vi "CreateSignals.vi"(8 "error in (no error)":errorcluster, 11 "DAQList in":refnum<class "DAQList.lvclass">) -> (0 "error out":errorcluster, 2 "Measurement Signals":refnum<k21>[](array[refnum]), 3 "DAQList out":refnum<class "DAQList.lvclass">)   [LabVIEW 2019, in "XCP_DaqDtoId.lvlib" / "DAQList.lvclass"]
uses:
  DAQList.lvclass
  DAQList.lvclass/DAQList.ctl
  <vilib>/ECUMC/ECUMC.llb/MC Get Prop Meas Address.vi
  <vilib>/xnet/xnet.llb/XNET Database Create (Signal).vi
  <vilib>/xnet/xnet.llb/XNET Database Create (Subframe).vi
  <vilib>/Utility/error.llb/Error Cluster From Error Code.vi
  <vilib>/ECUMC/ECUMC.llb/MC Get Prop Meas Data Type.vi
  TypeDef/Global.vi
  <vilib>/xnet/xnet.llb/XNET Database Create (Dynamic Signal).vi
  <vilib>/ECUMC/ECUMC.llb/MC Get Prop Meas Comment.vi
  <vilib>/ECUMC/ECUMC.llb/MC Get Prop Meas Scaling Offset.vi
  <vilib>/ECUMC/ECUMC.llb/MC Get Prop Meas Scaling Factor.vi
  <vilib>/ECUMC/ECUMC.llb/MC Get Prop Meas Minimum.vi
  <vilib>/ECUMC/ECUMC.llb/MC Get Prop Meas Maximum.vi
  <vilib>/ECUMC/ECUMC.llb/MC Get Prop Meas Byte Order.vi
  <vilib>/ECUMC/ECUMC.llb/MC Get Prop Meas Unit.vi
  <vilib>/ErrorRing/Error Ring.xnode
  <resource>/objmgr/xnet.rc
  <vilib>/ECUMC/ECUMC.lvlib
panel:
  out "Previous Offset":i32
  out "Previous Flag":bool
  out "Meas Split Addr Offset":i32
  out "Meas Split Flag":bool
  out "Search Addr":u32 format="%.0x"
  out "Latest Command Pair":u8[][](array[numeric]) format="%.0x"
  in  "For Loop Iteration":i32=-1 caption="#pairs to process (-1 for all)"
  out "Filtered Command Pairs":u8[][][](array[numeric]) format="%.0x"
  # "Debugging Panel"
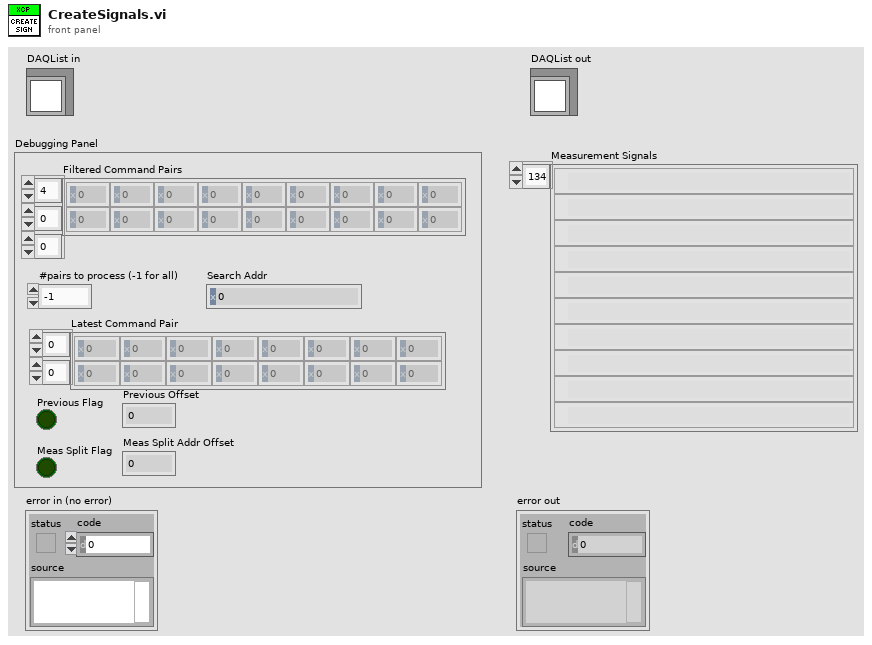
[diagram p1: front panel]
types:
  T1 = typedef "ECUMC.lvlib/MC Reference.ctt" = u32
  T2 = typedef "ECUMC.lvlib/MC Data Type.ctt" = u8
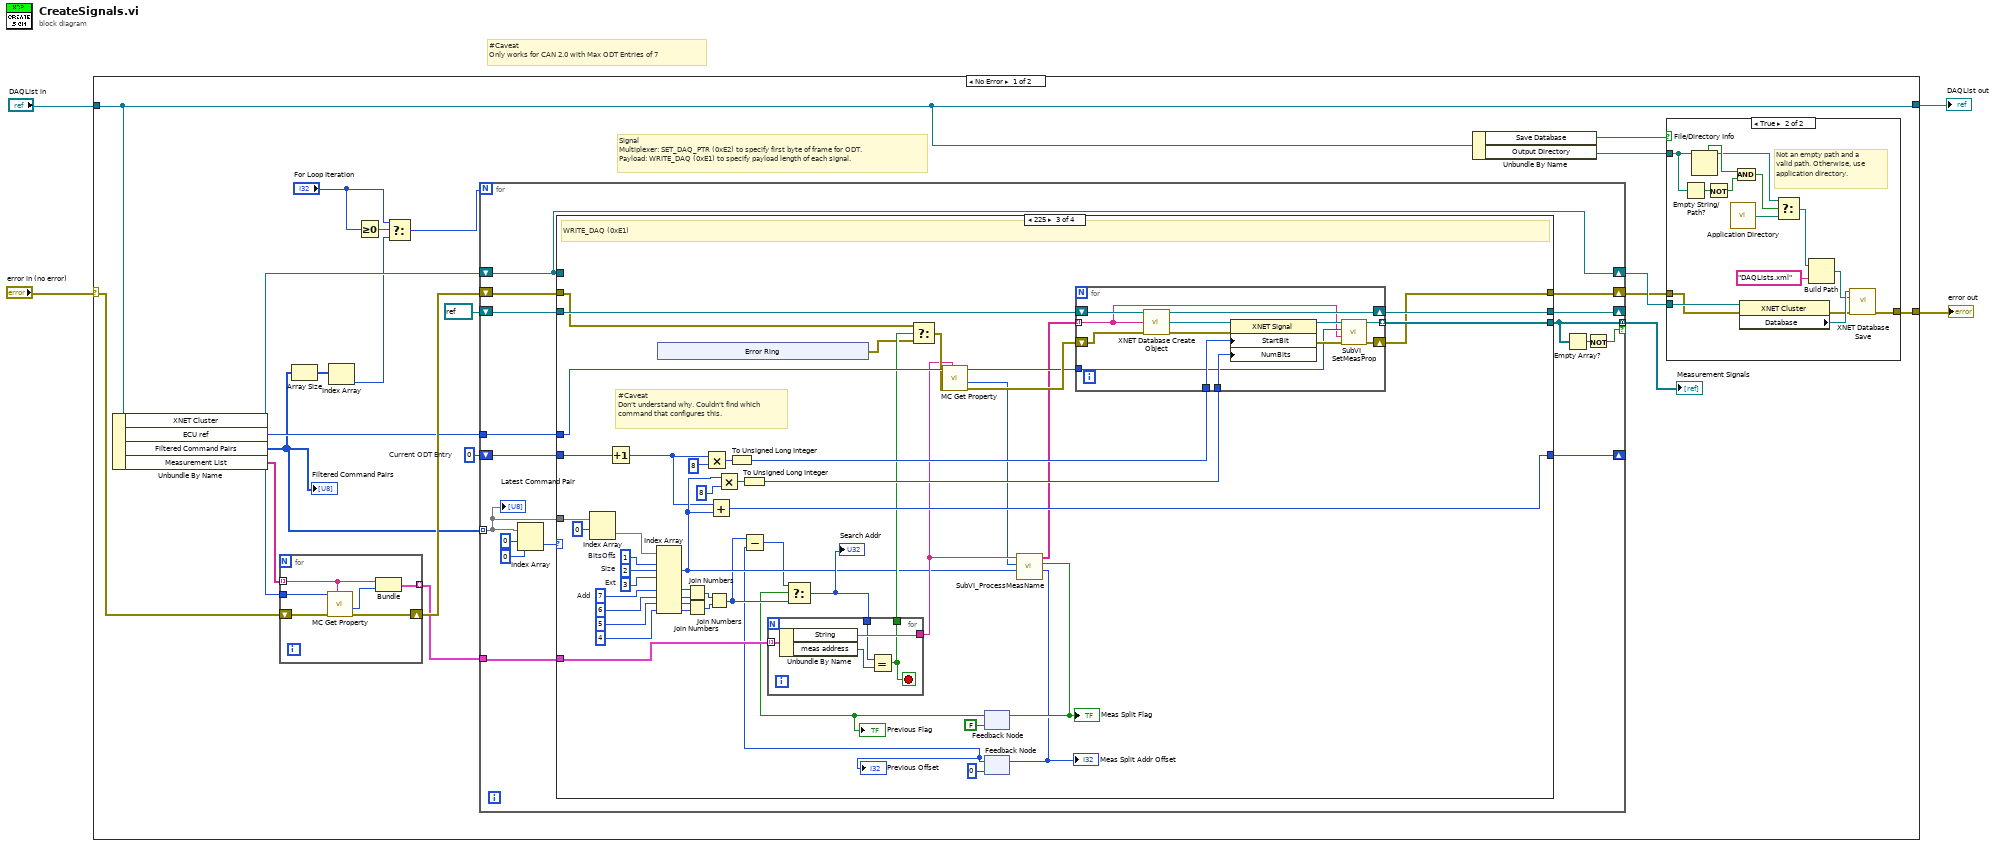
[diagram p0: block diagram]
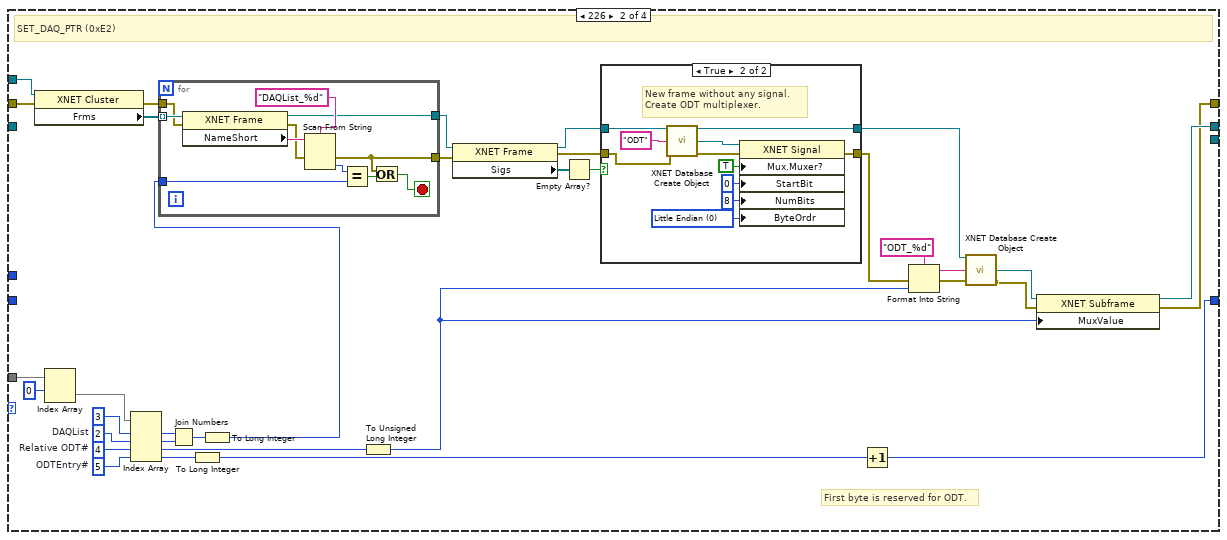
[diagram p3: hidden frame]
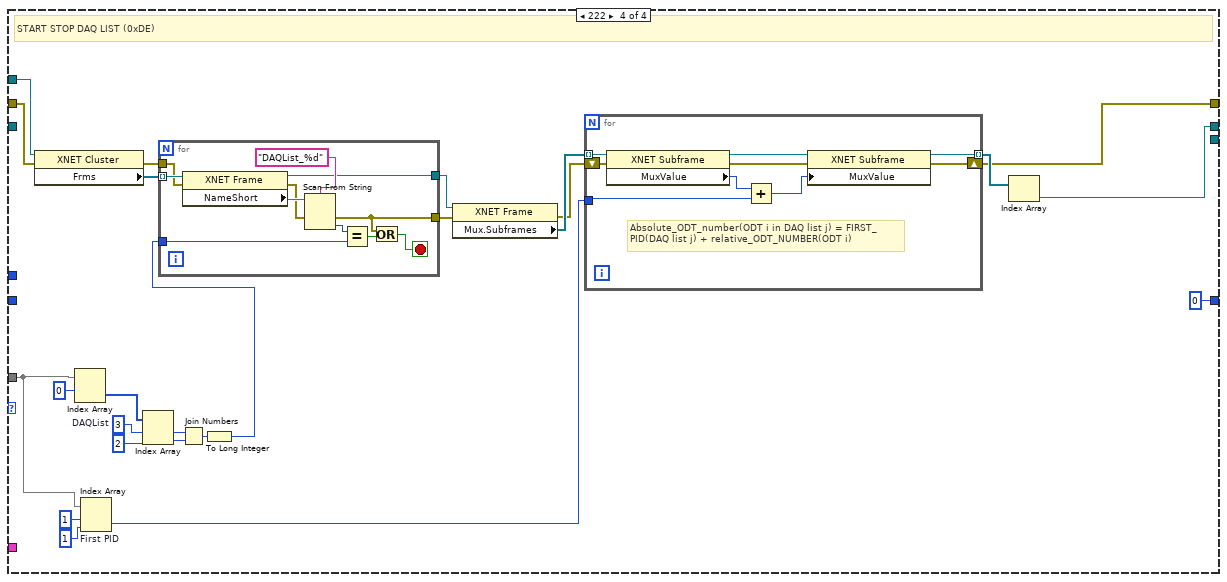
[diagram p5: hidden frame]
diagram:
  # "#Caveat\nOnly works for CAN 2.0 with Max ODT Entries of 7"
  n1 = case shown="No Error" "error in (no error)" {
    selector: "error in (no error)" -> [w19 w243]
    tunnel: [w18 w243] -> w3
    tunnel: [w16 w242] -> w1
    tunnel: "DAQList in" -> [w16 w242]
    frame No Error {
      w25 = 0  # Current ODT Entry
      # "Signal\nMultiplexer: SET_DAQ_PTR (0xE2) to specify first byte of frame for ODT.\nPayload: WRITE_DAQ (0xE1) to specify payload length of each signal."
      n2 = Unbundle By Name(w16) -> ("XNET Cluster"=w13:refnum<k21>, "ECU ref"=w22:T1, "Filtered Command Pairs"=w8:u8[][][], "Measurement List"=w12:string[])
      "Filtered Command Pairs" <- w8
      n3 = for {
        tunnel: w12 -> [w31] mode=indexing
        tunnel: w22 -> [w29]
        tunnel: [w27] -> w17 mode=indexing
        shift-right: [w26] -> w24
        shift-left: w19 -> [w28]
        n4 = call-poly <vilib>:"MC Get Property.vi"("name"=w31, "error in"=w28, "reference in"=w29) -> ("error out"=w26:errorcluster, "meas address"=w30:u32)  [unwired: 6 in, 1 out]
        n5 = Bundle("String"=w31, "meas address"=w30) -> (w27:cluster{"String":string, "meas address":u32})  [unwired: 1 in]
      }
      n6 = Array Size(array=w8) -> (size(s)=w6:i32[])
      n7 = Index Array(array=w6) -> (element=w5:i32)  [unwired: 1 in]
      n8 = Greater Or Equal To 0?(x="For Loop Iteration") -> (x >= 0?=w10:bool)
      n9 = Select(t="For Loop Iteration", s=w10, f=w5) -> (s? t:f=w9:i32)
      n10 = for {
        N: w9 -> [_]
        tunnel: w8 -> [w47] mode=indexing
        shift-right: [w42] -> _
        shift-left: w25 -> [w43]
        shift-right: [w40] -> w20
        shift-left: w24 -> [w41]
        shift-right: [w39] -> _
        shift-left: refnum<k21> refnum ("Mux.Subfrm") -> [w38]
        tunnel: w22 -> [w37]
        tunnel: w17 -> [w36]
        tunnel: [w34] -> w11 mode=concatenating if=w32
        shift-right: [w33] -> w21
        shift-left: w13 -> [w33]
        n11 = Index Array(array=w47, index (row)=0, index (col)=0 ("disabled index (col)")) -> (element=w44:u8)
        n12 = case shown="225" w44 {
          tunnel: w47 -> [_ w84 w154 w190]
          tunnel: w43 -> [w50 _ w134 _]
          tunnel: [w50 w71 w133 0 ("Current ODT Entry")] -> w42
          tunnel: w33 -> [_ w51 _ w182]
          tunnel: w41 -> [w49 w77 w125 w200]
          tunnel: [w49 w75 w128 w184] -> w40
          tunnel: [w48 w76 w135 w186] -> w39
          tunnel: w38 -> [w48 _ w152 _]
          tunnel: w37 -> [_ _ w132 _]
          tunnel: w36 -> [_ _ w136 _]
          tunnel: [_ _ w129 _] -> w34
          frame 0, Default {
            # "Do nothing."
          }
          frame 226 {
            w83 = 5  # ODTEntry#
            w82 = 4  # Relative ODT#
            w81 = 2  # DAQList
            # "First byte is reserved for ODT."
            # "SET_DAQ_PTR (0xE2)"
            n13 = property class="XNET Cluster"(reference=w51, error in=w77) -> (error out=w78:errorcluster, "Frms"=w79:refnum<k21>[])  [unwired: 1 out]
            n14 = Index Array(array=w84, index (row)=0) -> (element=w80:u8[])  [unwired: 1 in]
            n15 = Index Array(array=w80, index #1=3 ("index"), index #2=w81, index #3=w82, index #4=w83) -> (element #1=w54:u8, element #2=w53:u8, element #3=w56:u8, element #4=w73:u8)
            n16 = Join Numbers(hi=w54, lo=w53) -> ((hi.lo)=w52:u16)
            n17 = To Long Integer(number=w73) -> (32bit integer=w72:i32)
            n18 = To Long Integer(number=w52) -> (32bit integer=w74:i32)
            n19 = for {
              tunnel: w79 -> [w96] mode=indexing
              tunnel: w74 -> [w92]
              tunnel: w78 -> [w91]
              tunnel: [w89] -> w62
              tunnel: [w87] -> w61
              stop <- w86 stop-if-true
              n20 = property class="XNET Frame"(reference=w96, error in=w91) -> (reference out=w89:refnum<k21>, error out=w90:errorcluster, "NameShort"=w95:string)
              n21 = Scan From String(format string="DAQList_%d", input string=w95, error in=w90) -> (error out=w87:errorcluster, output 1=w93:i32)  [unwired: 2 in, 2 out]
              n22 = Equal?(x=w93, y=w92) -> (x = y?=w88:bool)
              n23 = Or(x=w87, y=w88) -> (x .or. y?=w86:bool)
            }
            n24 = To Unsigned Long Integer(number=w56) -> (unsigned 32bit integer=w68:u32)
            n25 = property class="XNET Frame"(reference=w62, error in=w61) -> (reference out=w60:refnum<k21>, error out=w57:errorcluster, "Sigs"=w59:refnum<k21>[])
            n26 = Empty Array?(array=w59) -> (empty?=w58:bool)
            n27 = case shown="True" w58 {
              tunnel: [w98 w103] -> w70
              tunnel: [w97 w102] -> w66
              tunnel: w60 -> [w98 w101]
              tunnel: w57 -> [w97 w99]
              frame False {
              }
              frame True {
                w104 = u32 0 items=["Little Endian", "Big Endian"] ("Byte Order")
                # "New frame without any signal.\nCreate ODT multiplexer."
                n28 = call-poly <vilib>:"XNET Database Create Object.vi"("frame in"=w101, "signal name"="ODT", "error in (no error)"=w99) -> ("frame out"=w103:refnum<k21>, "signal out"=w109:refnum<k21>, "error out"=w108:errorcluster)  [unwired: 10 in]
                n29 = property class="XNET Signal"(reference=w109, error in=w108, "Mux.Muxer?"=TRUE ("Mux:Data Multiplexer?"), "StartBit"=u32 0 ("Start Bit"), "NumBits"=u32 8 ("Number of Bits"), "ByteOrdr"=w104) -> (error out=w102:errorcluster)  [unwired: 1 out]
              }
            }
            n30 = Increment(x=w72) -> (x+1=w71:i32)
            n31 = Format Into String(format string="ODT_%d", error in=w66, w68) -> (resulting string=w67:string, error out=w65:errorcluster)  [unwired: 1 in]
            n32 = call-poly <vilib>:"XNET Database Create Object.vi"("frame in"=w70, "subframe name"=w67, "error in (no error)"=w65) -> ("subframe out"=w63:refnum<k21>, "error out"=w64:errorcluster)  [unwired: 10 in, 1 out]
            n33 = property class="XNET Subframe"(reference=w63, error in=w64, "MuxValue"=w68) -> (reference out=w76:refnum<k21>, error out=w75:errorcluster)
          }
          frame 225 {
            w153 = 7  # Add
            w158 = 3  # Ext
            w157 = 2  # Size
            w156 = 1  # BitsOffs
            # "#Caveat\nDon't understand why. Couldn't find which command that configures this."
            # "WRITE_DAQ (0xE1)"
            n34 = Index Array(array=w154, index (row)=0) -> (element=w155:u8[])  [unwired: 1 in]
            n35 = Increment(x=w134) -> (x+1=w110:i32)
            n36 = Index Array(array=w155, index #1=w156, index #2=w157, index #3=w158, index #5=w153, index #6=6 ("index"), index #7=5 ("index"), index #8=4 ("index")) -> (element #2=w119:u8, element #5=w142:u8, element #6=w141:u8, element #7=w140:u8, element #8=w139:u8)  [unwired: 1 in, 3 out]
            n37 = xnode "Error Ring"() -> ("error out"=w123:errorcluster)
            n38 = Join Numbers(hi=w142, lo=w141) -> ((hi.lo)=w137:u16)
            n39 = Join Numbers(hi=w140, lo=w139) -> ((hi.lo)=w138:u16)
            n40 = Multiply(x=w110, y=8) -> (x*y=w151:i32)
            n41 = Join Numbers(hi=w137, lo=w138) -> ((hi.lo)=w118:u32)
            n42 = Add(x=w110, y=w119) -> (x+y=w133:i32)
            n43 = Multiply(x=w119, y=u8 8) -> (x*y=w147:u8)
            n44 = To Unsigned Long Integer(number=w151) -> (unsigned 32bit integer=w149:u32)
            n45 = To Unsigned Long Integer(number=w147) -> (unsigned 32bit integer=w146:u32)
            n46 = feedback #1(FALSE ("Meas Split Flag")) -> (w116:bool)
            "Previous Flag" <- w116
            n47 = feedback #2(0 ("Add Offset")) -> (w114:i32)
            "Previous Offset" <- w114
            n48 = Subtract(x=w118, y=w114) -> (x-y=w117:u32)
            n49 = Select(t=w117, s=w116, f=w118) -> (s? t:f=w130:u32)
            "Search Addr" <- w130
            n50 = for {
              tunnel: w136 -> [w181] mode=indexing
              tunnel: w130 -> [w178]
              tunnel: [w180] -> w122
              tunnel: [w177] -> w126
              stop <- w177 stop-if-true
              n51 = Unbundle By Name(w181) -> ("String"=w180:string, "meas address"=w179:u32)
              n52 = Equal?(x=w178, y=w179) -> (x = y?=w177:bool)
            }
            n53 = Select(t=w125, s=w126, f=w123) -> (s? t:f=w124:errorcluster)
            n54 = call-poly <vilib>:"MC Get Property.vi"("name"=w122, "error in"=w124, "reference in"=w132) -> ("error out"=w131:errorcluster, "meas data type"=w120:T2, "reference out"=w127:T1)  [unwired: 6 in]
            n55 = call "SubVI_ProcessMeasName.vi"("Write DAQ Size"=w119, "meas data type"=w120, "Meas Name"=w122) -> ("Meas Split Addr Offset"=w113:i32, "Meas Split Flag"=w115:bool, "DAQ List Signal Name"=w121:string[])  [unwired: 6 in]
            "Meas Split Flag" <- w115
            "Meas Split Addr Offset" <- w113
            n56 = feedback-in #1(w115) -> ()
            n57 = feedback-in #2(w113) -> ()
            n58 = for {
              tunnel: w149 -> [w170]
              tunnel: w146 -> [w169]
              tunnel: [w164] -> w129 mode=indexing
              tunnel: w127 -> [w161]
              shift-right: [w167] -> w135
              shift-left: w152 -> [w172]
              shift-right: [w162] -> w128
              shift-left: w131 -> [w166]
              tunnel: w121 -> [w160] mode=indexing
              n59 = call-poly <vilib>:"XNET Database Create Object.vi"("subframe in"=w172, "signal name"=w160, "error in (no error)"=w166) -> ("subframe out"=w167:refnum<k21>, "signal out"=w171:refnum<k21>, "error out"=w168:errorcluster)  [unwired: 10 in]
              n60 = property class="XNET Signal"(reference=w171, error in=w168, "StartBit"=w170, "NumBits"=w169) -> (reference out=w165:refnum<k21>, error out=w163:errorcluster)
              n61 = call "SubVI_SetMeasProp.vi"("error in"=w163, "Signal Name"=w160, "ECU Ref"=w161, "XNET Signal In"=w165) -> ("error out"=w162:errorcluster, "XNET Signal Out"=w164:refnum<k21>)  [unwired: 6 in]
            }
          }
          frame 222 {
            w204 = 3  # DAQList
            # "START STOP DAQ LIST (0xDE)"
            n62 = property class="XNET Cluster"(reference=w182, error in=w200) -> (error out=w201:errorcluster, "Frms"=w202:refnum<k21>[])  [unwired: 1 out]
            n63 = Index Array(array=w190, index (row)=0) -> (element=w203:u8[])  [unwired: 1 in]
            n64 = Index Array "First PID"(array=w190, index (row)=1, index (col)=1 ("disabled index (col)")) -> (element=w183:u8)
            n65 = Index Array(array=w203, index #1=w204, index #2=2 ("index")) -> (element #1=w195:u8, element #2=w194:u8)
            n66 = Join Numbers(hi=w195, lo=w194) -> ((hi.lo)=w193:u16)
            n67 = To Long Integer(number=w193) -> (32bit integer=w192:i32)
            n68 = for {
              tunnel: w202 -> [w216] mode=indexing
              tunnel: w192 -> [w212]
              tunnel: w201 -> [w211]
              tunnel: [w209] -> w199
              tunnel: [w207] -> w198
              stop <- w206 stop-if-true
              n69 = property class="XNET Frame"(reference=w216, error in=w211) -> (reference out=w209:refnum<k21>, error out=w210:errorcluster, "NameShort"=w215:string)
              n70 = Scan From String(format string="DAQList_%d", input string=w215, error in=w210) -> (error out=w207:errorcluster, output 1=w213:i32)  [unwired: 2 in, 2 out]
              n71 = Equal?(x=w213, y=w212) -> (x = y?=w208:bool)
              n72 = Or(x=w207, y=w208) -> (x .or. y?=w206:bool)
            }
            n73 = property class="XNET Frame"(reference=w199, error in=w198) -> (error out=w187:errorcluster, "Mux.Subframes"=w191:refnum<k21>[])  [unwired: 1 out]
            n74 = for {
              tunnel: w191 -> [w225] mode=indexing
              tunnel: [w221] -> w185 mode=indexing
              shift-right: [w220] -> w184
              shift-left: w187 -> [w224]
              tunnel: w183 -> [w218]
              # "Absolute_ODT_number(ODT i in DAQ list j) = FIRST_PID(DAQ list j) + relative_ODT_NUMBER(ODT i)"
              n75 = property class="XNET Subframe"(reference=w225, error in=w224) -> (reference out=w223:refnum<k21>, error out=w222:errorcluster, "MuxValue"=w219:u32)
              n76 = Add(x=w219, y=w218) -> (x+y=w217:u32)
              n77 = property class="XNET Subframe"(reference=w223, error in=w222, "MuxValue"=w217) -> (reference out=w221:refnum<k21>, error out=w220:errorcluster)
            }
            n78 = Index Array(array=w185) -> (element=w186:refnum<k21>)  [unwired: 1 in]
          }
        }
        n79 = Empty Array?(array=w34) -> (empty?=w35:bool)
        n80 = Not(x=w35) -> (.not. x?=w32:bool)
        "Latest Command Pair" <- w47
      }
      "Measurement Signals" <- w11
      n81 = Unbundle By Name(w16) -> ("Save Database"=w15:bool, "Output Directory"=w14:path)
      n82 = case shown="True" w15 {
        tunnel: [w226 w227] -> w18
        tunnel: w21 -> [_ w239]
        tunnel: w20 -> [w226 w238]
        tunnel: w14 -> [_ w235]
        frame False {
        }
        frame True {
          # "Not an empty path and a valid path. Otherwise, use application directory."
          n83 = Empty String/Path?(string/path=w235) -> (empty?=w233:bool)
          n84 = File/Directory Info(path=w235) -> (path out=w230:path, directory=w234:bool)  [unwired: 1 in, 5 out]
          n85 = Not(x=w233) -> (.not. x?=w232:bool)
          n86 = call <vilib>:"Application Directory.vi"() -> ("Application Directory"=w229:path)
          n87 = And(x=w234, y=w232) -> (x .and. y?=w231:bool)
          n88 = property class="XNET Cluster"(reference=w239, error in=w238) -> (error out=w228:errorcluster, "Database"=w240:refnum<k21>)  [unwired: 1 out]
          n89 = Select(t=w230, s=w231, f=w229) -> (s? t:f=w237:path)
          n90 = Build Path(base path=w237, name or relative path="DAQLists.xml") -> (appended path=w236:path)
          n91 = call <vilib>:"XNET Database Save.vi"("database in"=w240, "filepath (empty)"=w236, "error in (no error)"=w228) -> ("error out"=w227:errorcluster)  [unwired: 11 in, 1 out]
        }
      }
    }
    frame Error {
    }
  }
  "error out" <- w3
  "DAQList out" <- w1
